vi "Init.vi"(8 "error in (no error)":errorcluster, 10 "Name":string, 11 "Process In":refnum<class "Debug Process.lvclass">) -> (0 "error out":errorcluster, 3 "Process Out":refnum<class "Debug Process.lvclass">)   [LabVIEW 2020, in "Debug Process.lvclass"]
doc: "Initializes the process and creates necessary references. Anything initialized here is released in the Clear.vi method."
uses:
  Debug Process.lvclass
  Debug Process.lvclass/Debug Process.ctl
  Protected/Broadcasting/Broadcast Message Cluster.ctl
  Public/Lifecycle/Lifecycle State.ctl
  Protected/Messaging/Message Cluster.ctl
  Protected/Messaging/Request Message Cluster.ctl
  <vilib>/Utility/error.llb/Clear Errors.vi
  <vilib>/Utility/error.llb/Error Cluster From Error Code.vi
  <vilib>/ErrorRing/Error Ring.xnode
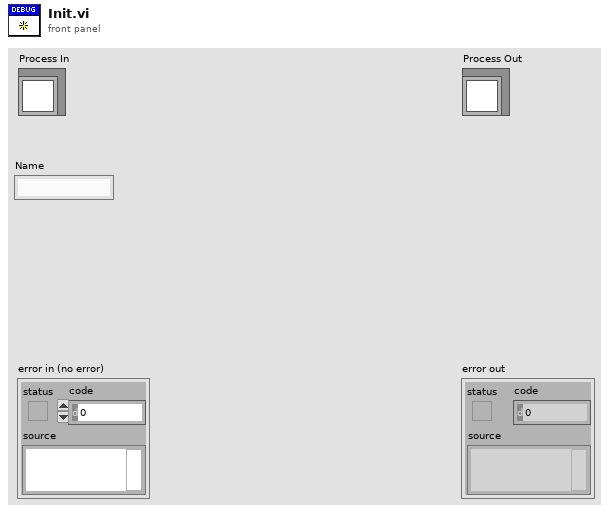
[diagram p1: front panel]
types:
  T1 = typedef "Debug Process.lvclass/Lifecycle State.ctl" = enum16{"Uninitialized", "Initialized", "Started", "Running", "Stopped", "Finished"}
  T2 = typedef "Debug Process.lvclass/Broadcast Message Cluster.ctl" = cluster{"Sender":string, "Message":string, "Message Data":variant}
  T3 = typedef "Debug Process.lvclass/Message Cluster.ctl" = cluster{"Message":string, "Message Data":variant, "Request Notifier":refnum<notifier>}
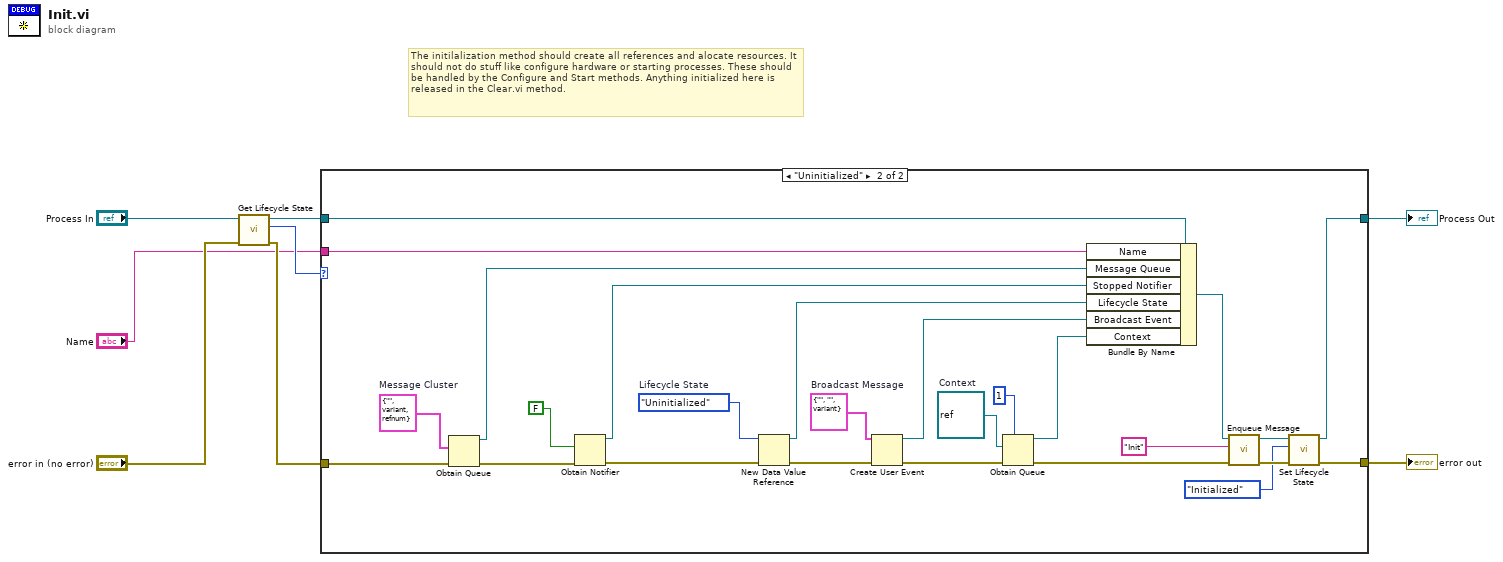
[diagram p0: block diagram]
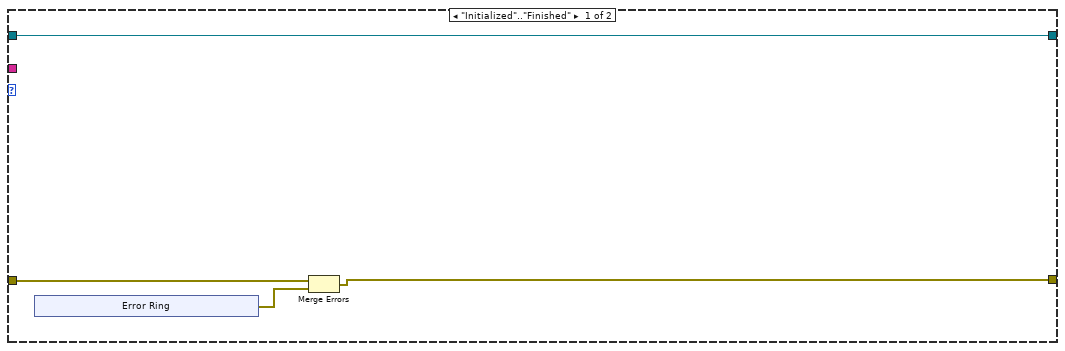
[diagram p2: hidden frame]
diagram:
  # "The initilalization method should create all references and alocate resources. It should not do stuff like configure hardware or starting processes. These should be handled by the Configure and Start methods. Anything initialized here is released in the Clear.vi method."
  n1 = call "Get Lifecycle State.vi"("error in (no error)"="error in (no error)", "Process In"="Process In") -> ("error out"=w3:errorcluster, "Lifecycle State"=w7:T1, "Process Out"=w8:refnum<class "Debug Process.lvclass">)  [unwired: 6 in, 1 out]
  n2 = case shown="\"Uninitialized\"" w7 {
    tunnel: [w12 w36] -> w6
    tunnel: [w9 w33] -> w5
    tunnel: w8 -> [w12 w28]
    tunnel: w3 -> [w10 w27]
    tunnel: "Name" -> [_ w17]
    frame "Initialized".."Finished" {
      n3 = xnode "Error Ring"() -> ("error out"=w11:errorcluster)
      n4 = Merge Errors(w10, w11) -> (w9:errorcluster)
    }
    frame "Uninitialized" {
      w22 = refnum<class> refnum  # Context
      w26 = T2 {"Sender"="", "Message"="", "Message Data"=variant}  # Broadcast Message
      w38 = Lifecycle_State."Uninitialized"  # Lifecycle State
      w32 = T3 {"Message"="", "Message Data"=variant, "Request Notifier"=refnum}  # Message Cluster
      n5 = Obtain Queue(element data type=w32, error in (no error)=w27) -> (queue out=w42:refnum<queue>, error out=w31:errorcluster)  [unwired: 3 in, 1 out]
      n6 = Obtain Notifier(notification data type=FALSE, error in (no error)=w31) -> (notifier out=w18:refnum<notifier>, error out=w39:errorcluster)  [unwired: 2 in, 1 out]
      n7 = New Data Value Reference(data value=w38, error in=w39) -> (data value reference=w37:refnum<data-value>, error out=w29:errorcluster)
      n8 = Create User Event(user event datatype=w26, error in=w29) -> (user event=w25:refnum<user-event>, error out=w24:errorcluster)
      n9 = Obtain Queue(max queue size (-1, unlimited)=1, element data type=w22, error in (no error)=w24) -> (queue out=w20:refnum<queue>, error out=w23:errorcluster)  [unwired: 2 in, 1 out]
      n10 = Bundle By Name(cluster=w28, "Name"=w17, "Message Queue"=w42, "Stopped Notifier"=w18, "Lifecycle State"=w37, "Broadcast Event"=w25, "Context"=w20) -> (w30:refnum<class "Debug Process.lvclass">)
      n11 = call "Enqueue Message.vi"("error in (no error)"=w23, "Message"="Init", "Process In"=w30) -> ("error out"=w35:errorcluster, "Process Out"=w41:refnum<class "Debug Process.lvclass">)  [unwired: 7 in]
      n12 = call "Set Lifecycle State.vi"("error in (no error)"=w35, "Lifecycle State"=Lifecycle_State."Initialized", "Process In"=w41) -> ("error out"=w33:errorcluster, "Process Out"=w36:refnum<class "Debug Process.lvclass">)  [unwired: 7 in]
    }
  }
  "error out" <- w5
  "Process Out" <- w6
